vi "ClearColumnOf2DArrayCtrl.vi"(10 "차원 크기":i32, 11 "ref array in":refnum<vi>) -> (3 "ref array out":refnum<vi>)   [LabVIEW 2018, in "Library-Ctrl.lvlib"]
uses:
  Library-Ctrl.lvlib
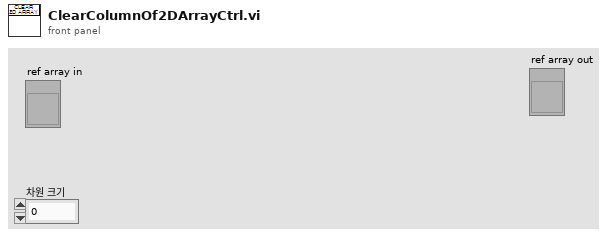
[diagram p1: front panel]
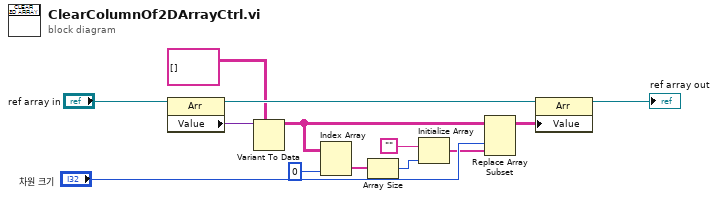
[diagram p0: block diagram]
diagram:
  n1 = property class="Arr"(reference="ref array in") -> (reference out=w11:refnum<vi>, "Value"=w12:variant)  [unwired: 1 in, 1 out]
  n2 = Variant To Data(type=string[][] [], Variant=w12) -> (data=w3:string[][])  [unwired: 1 in, 1 out]
  n3 = Index Array(array=w3, index (col)=0 ("인덱스 (행)")) -> (element=w6:string[])  [unwired: 1 in]
  n4 = Array Size(array=w6) -> (size(s)=w5:i32)
  n5 = Initialize Array("", w5) -> (w2:string[])
  n6 = Replace Array Subset(array=w3, new element=w2, index (col)="차원 크기") -> (w10:string[][])  [unwired: 1 in]
  n7 = property class="Arr"(reference=w11, "Value"=w10) -> (reference out=→"ref array out":refnum<vi>)  [unwired: 1 in, 1 out]
